vi "Filter Test.vi"() -> ()   [LabVIEW 2015]
uses:
  Controls/Filter XCtl/Filter XCtl.xctl
  Utility VIs/Math VIs/Linear to dB (array).vi
panel:
  out "Magnitude":dbl[](graph)
  in  "Sampling rate (Hz)":dbl=100000.0
  in  "Quadrature":bool
  in  "Filter":T1(xcontrol)
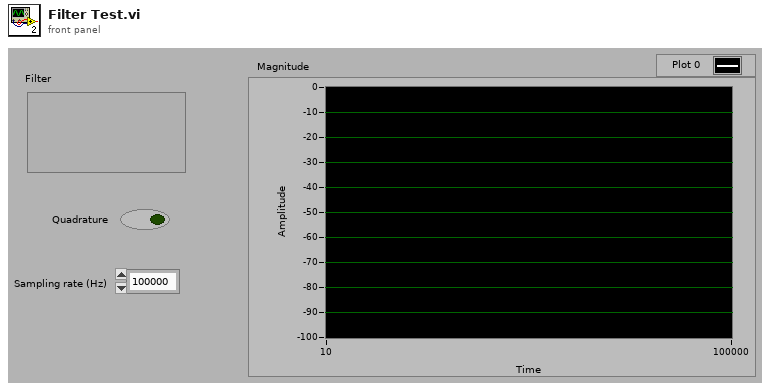
[diagram p1: front panel]
types:
  T1 = cluster{"CF (kHz)":dbl, "BW (kHz)":dbl, "IIR Filter Cluster":cluster{"filter structure":enum32{"IIR 2nd Order", "IIR 4th Order"}, "Reverse Coefficients":dbl[], "Forward Coefficients":dbl[]}, "Final Filter State":dbl[], "Scale Factor":dbl, "Final Filter State 2":dbl[], "Quadrature":bool, "Type":enum16{"Lowpass", "Highpass", "Bandpass", "Bandstop", "OFF"}}
  T2 = typedef "Filter XCtl.xctl/Filter Data.ctl" = cluster{"CF (kHz)":dbl, "BW (kHz)":dbl, "IIR Filter Cluster":cluster{"filter structure":enum32{"IIR 2nd Order", "IIR 4th Order"}, "Reverse Coefficients":dbl[], "Forward Coefficients":dbl[]}, "Final Filter State":dbl[], "Scale Factor":dbl, "Final Filter State 2":dbl[], "Quadrature":bool, "Type":enum16{"Lowpass", "Highpass", "Bandpass", "Bandstop", "OFF"}}
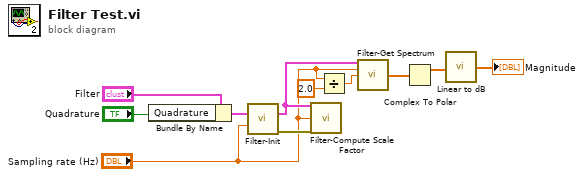
[diagram p0: block diagram]
diagram:
  n1 = Bundle By Name(cluster="Filter", "Quadrature"="Quadrature") -> (w9:T1)
  n2 = call "Filter-Init.vi"("Filter"=w9, "Sampling rate (Hz)"="Sampling rate (Hz)") -> ("Filter out"=w7:T2, "error out"=w8:errorcluster)  [unwired: 12 in]
  n3 = call "Filter-Compute Scale Factor.vi"("Filter"=w7, "Sampling Rate (Hz)"="Sampling rate (Hz)", "error in (no error)"=w8) -> ()  [unwired: 11 in, 2 out]
  n4 = Divide(x="Sampling rate (Hz)", y=2.0) -> (x/y=w6:dbl)
  n5 = call "Filter-Get Spectrum.vi"("Filter"=w7, "Sampling Rate (Hz)"="Sampling rate (Hz)", "Npts"=w6) -> ("spectrum"=w3:cdb[])  [unwired: 10 in, 2 out]
  n6 = Complex To Polar(r * e^(i*theta)=w3) -> (r=w2:dbl[])  [unwired: 1 out]
  n7 = call-poly "Linear to dB.vi"("linear"=w2) -> ("dB"=→"Magnitude":dbl[])
